vi "Init_ENET.vi"(3 "error in (no error)":errorcluster, 5 "Num do ASRL do Enet":string="1") -> (0 "ENET error out":errorcluster, 2 "ENET resource name":refnum<visa-resource-name>)   [LabVIEW 2012]
uses:
  <vilib>/Instr/_visa.llb/VISA Configure Serial Port (Instr).vi
panel:
  in  "VISA session (for class)":refnum<visa-resource-name>
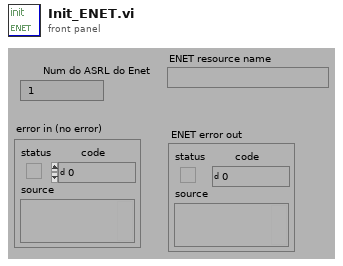
[diagram p1: front panel]
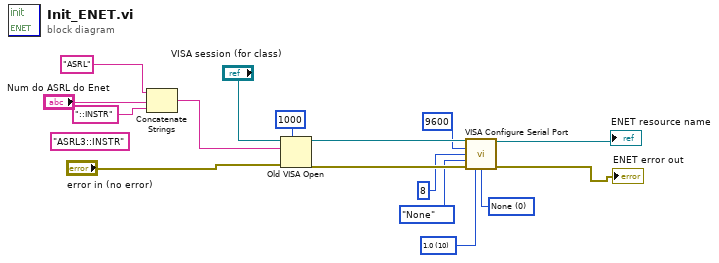
[diagram p0: block diagram]
diagram:
  w2 = u16 0 items=["None", "XON/XOFF", "RTS/CTS", "XON/XOFF & RTS/CTS", "DTR/DSR", "XON/XOFF & DTR/DSR"] ("flow control (0:none)")
  w3 = u16 10 items=["1.0"=10, "1.5"=15, "2.0"=20] ("stop bits (10: 1 bit)")
  (unwired) "ASRL3::INSTR" ("resource name (\"\")")
  n1 = Concatenate Strings("ASRL", "Num do ASRL do Enet", "::INSTR" ("string")) -> (w11:string)
  n2 = Old VISA Open(7:u32 1000 ("VISA Open timeout (0)"), 8:"error in (no error)", 10:w11, 11:"VISA session (for class)") -> (0:w7:errorcluster, 3:w10:refnum<visa-resource-name>)  [unwired: 1 in]
  n3 = call-poly "VISA Configure Serial Port"("VISA resource name"=w10, "baud rate (9600)"=u32 9600, "data bits (8)"=u16 8, "parity (0:none)"=enum16{"None", "Odd", "Even", "Mark", "Space"}."None", "error in (no error)"=w7, "stop bits (10: 1 bit)"=w3, "flow control (0:none)"=w2) -> ("VISA resource name out"=→"ENET resource name":refnum<visa-resource-name>, "error out"=→"ENET error out":errorcluster)  [unwired: 7 in]
